vi "Open Drive Motors.vi"(5 "Open Butterfly Drive?":bool, 6 "Idle Mode":T1, 7 "Set Master/Follower?":bool, 9 "CAN IDs":u8[](array[numeric]), 11 "Full Acceleration Time":sgl) -> ()   [LabVIEW 2018]
uses:
  <vilib>/Rock Robotics/WPI/ThirdParty/REV Robotics/SPARK MAX/Typedef/Spark MAX Idle Mode.ctl
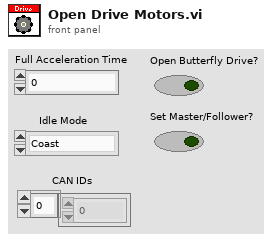
[diagram p1: front panel]
types:
  T1 = typedef "Spark MAX Idle Mode.ctl" = enum16{"Coast", "Brake"}
  T2 = typedef "WPI_MotorControlDeviceRef.ctl" = cluster{"DeviceStatus":errorcluster, "Type":T3, "PWM":cluster{"PWM Channel":T4, "DeadBand":T5}, "CAN":cluster{"Device Number":u8, "SetOutput VI Ref":variant, "GetOutput VI Ref":variant, "Enable VI Ref":variant, "Disable VI Ref":variant, "Data":variant}, "Invert":bool, "DIO PWM":cluster{"PWM \"Enable\" Channel":T4, "DIOChannel":T6, "PWM Rate":dbl}}
  T3 = typedef "WPI_MotorControlType.ctl" = enum16{"PWM", "CAN", "DIO PWM"}
  T4 = typedef "FPGA_DIOPWMChannel.ctl" = enum8{"PWM 0", "PWM 1", "PWM 2", "PWM 3", "PWM 4", "PWM 5", "PWM 6", "PWM 7", "PWM 8", "PWM 9", "PWM MXP 0", "PWM MXP 1", "PWM MXP 2", "PWM MXP 3", "PWM MXP 4", "PWM MXP 5", "PWM MXP 6", "PWM MXP 7", "PWM MXP 8", "PWM MXP 9", "Invalid"}
  T5 = typedef "WPI_PWMDeadband.ctl" = cluster{"Name":string, "maxPositivePwm":i32, "minPositivePwm":i32, "centerPwm":i32, "maxNegativePwm":i32, "minNegativePwm":i32, "angularRange":u16}
  T6 = typedef "FPGA_DIOChannel.ctl" = enum8{"DIO 0", "DIO 1", "DIO 2", "DIO 3", "DIO 4", "DIO 5", "DIO 6", "DIO 7", "DIO 8", "DIO 9", "DIO MXP 0", "DIO MXP 1", "DIO MXP 2", "DIO MXP 3", "DIO MXP 4", "DIO MXP 5", "DIO MXP 6", "DIO MXP 7", "DIO MXP 8", "DIO MXP 9", "DIO MXP 10", "DIO MXP 11", "DIO MXP 12", "DIO MXP 13", "DIO MXP 14", "DIO MXP 15", "SPI Port CS1", "SPI Port CS2", "SPI Port CS3", "SPI Port MISO", "SPI Port MOSI", "Invalid"}
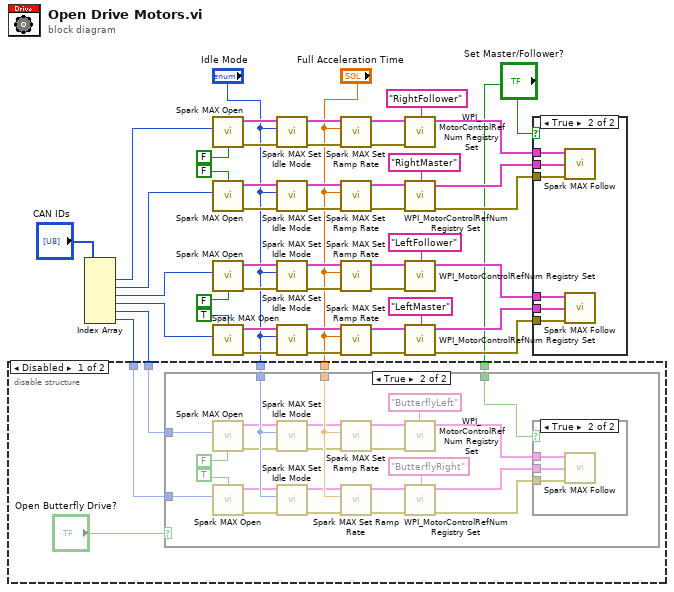
[diagram p0: block diagram]
diagram:
  n1 = Index Array(array="CAN IDs") -> (element #1=w10:u8, element #2=w9:u8, element #3=w8:u8, element #4=w7:u8, element #5=w6:u8, element #6=w5:u8)  [unwired: 6 in]
  n2 = disable-structure shown="Disabled" {
    disable-tunnel: w6 -> [w54 _]
    disable-tunnel: w5 -> [w53 _]
    disable-tunnel: "Full Acceleration Time" -> [w52 _]
    disable-tunnel: "Idle Mode" -> [w51 _]
    disable-tunnel: "Set Master/Follower?" -> [w49 _]
    frame Disabled {
      n3 = case shown="True" "Open Butterfly Drive?" {
        tunnel: w54 -> [_ w78]
        tunnel: w53 -> [_ w77]
        tunnel: w52 -> [_ w76]
        tunnel: w51 -> [_ w75]
        tunnel: w49 -> [_ w55]
        frame False {
        }
        frame True {
          n4 = call <vilib>:"Spark MAX Open.vi"("Invert"=FALSE, "Device Number"=w78) -> ("error out"=w59:errorcluster, "MotorControlDeviceRef"=w61:T2)  [unwired: 8 in]
          n5 = call <vilib>:"Spark MAX Open.vi"("Invert"=TRUE, "Device Number"=w77) -> ("error out"=w58:errorcluster, "MotorControlDeviceRef"=w60:T2)  [unwired: 8 in]
          n6 = call <vilib>:"Spark MAX Set Idle Mode.vi"("error in (no error)"=w59, "Idle Mode"=w75, "MotorControlDeviceRef in"=w61) -> ("error out"=w67:errorcluster, "MotorControlDeviceRef out"=w68:T2)  [unwired: 7 in]
          n7 = call <vilib>:"Spark MAX Set Idle Mode.vi"("error in (no error)"=w58, "Idle Mode"=w75, "MotorControlDeviceRef in"=w60) -> ("error out"=w65:errorcluster, "MotorControlDeviceRef out"=w69:T2)  [unwired: 7 in]
          n8 = call <vilib>:"Spark MAX Set Ramp Rate.vi"("error in (no error)"=w67, "Seconds from neutral to full (0)"=w76, "MotorControlDeviceRef in"=w68) -> ("error out"=w66:errorcluster, "MotorControlDeviceRef"=w70:T2)  [unwired: 7 in]
          n9 = call <vilib>:"Spark MAX Set Ramp Rate.vi"("error in (no error)"=w65, "Seconds from neutral to full (0)"=w76, "MotorControlDeviceRef in"=w69) -> ("error out"=w64:errorcluster, "MotorControlDeviceRef"=w71:T2)  [unwired: 7 in]
          n10 = call <vilib>:"WPI_MotorControlRefNum Registry Set.vi"("error in (no error)"=w66, "refnum name"="ButterflyLeft", "MotorControlDevRef"=w70) -> ("MotorControlDevRef"=w74:T2)  [unwired: 7 in, 1 out]
          n11 = call <vilib>:"WPI_MotorControlRefNum Registry Set.vi"("error in (no error)"=w64, "refnum name"="ButterflyRight", "MotorControlDevRef"=w71) -> ("error out"=w72:errorcluster, "MotorControlDevRef"=w73:T2)  [unwired: 7 in]
          n12 = case shown="True" w55 {
            tunnel: w74 -> [_ w81]
            tunnel: w73 -> [_ w80]
            tunnel: w72 -> [_ w79]
            frame False {
            }
            frame True {
              n13 = call <vilib>:"Spark MAX Follow.vi"("error in (no error)"=w79, "Master Controller"=w80, "MotorControlDeviceRef"=w81) -> ()  [unwired: 7 in, 2 out]
            }
          }
        }
      }
    }
    frame Enabled {
    }
  }
  n14 = call <vilib>:"Spark MAX Open.vi"("Invert"=FALSE, "Device Number"=w10) -> ("error out"=w35:errorcluster, "MotorControlDeviceRef"=w40:T2)  [unwired: 8 in]
  n15 = call <vilib>:"Spark MAX Open.vi"("Invert"=FALSE, "Device Number"=w9) -> ("error out"=w33:errorcluster, "MotorControlDeviceRef"=w39:T2)  [unwired: 8 in]
  n16 = call <vilib>:"Spark MAX Open.vi"("Invert"=FALSE, "Device Number"=w8) -> ("error out"=w31:errorcluster, "MotorControlDeviceRef"=w41:T2)  [unwired: 8 in]
  n17 = call <vilib>:"Spark MAX Open.vi"("Invert"=TRUE, "Device Number"=w7) -> ("error out"=w29:errorcluster, "MotorControlDeviceRef"=w42:T2)  [unwired: 8 in]
  n18 = call <vilib>:"Spark MAX Set Idle Mode.vi"("error in (no error)"=w35, "Idle Mode"="Idle Mode", "MotorControlDeviceRef in"=w40) -> ("error out"=w34:errorcluster, "MotorControlDeviceRef out"=w37:T2)  [unwired: 7 in]
  n19 = call <vilib>:"Spark MAX Set Idle Mode.vi"("error in (no error)"=w33, "Idle Mode"="Idle Mode", "MotorControlDeviceRef in"=w39) -> ("error out"=w32:errorcluster, "MotorControlDeviceRef out"=w38:T2)  [unwired: 7 in]
  n20 = call <vilib>:"Spark MAX Set Idle Mode.vi"("error in (no error)"=w31, "Idle Mode"="Idle Mode", "MotorControlDeviceRef in"=w41) -> ("error out"=w26:errorcluster, "MotorControlDeviceRef out"=w44:T2)  [unwired: 7 in]
  n21 = call <vilib>:"Spark MAX Set Idle Mode.vi"("error in (no error)"=w29, "Idle Mode"="Idle Mode", "MotorControlDeviceRef in"=w42) -> ("error out"=w28:errorcluster, "MotorControlDeviceRef out"=w43:T2)  [unwired: 7 in]
  n22 = call <vilib>:"Spark MAX Set Ramp Rate.vi"("error in (no error)"=w34, "Seconds from neutral to full (0)"="Full Acceleration Time", "MotorControlDeviceRef in"=w37) -> ("error out"=w24:errorcluster, "MotorControlDeviceRef"=w46:T2)  [unwired: 7 in]
  n23 = call <vilib>:"Spark MAX Set Ramp Rate.vi"("error in (no error)"=w32, "Seconds from neutral to full (0)"="Full Acceleration Time", "MotorControlDeviceRef in"=w38) -> ("error out"=w25:errorcluster, "MotorControlDeviceRef"=w45:T2)  [unwired: 7 in]
  n24 = call <vilib>:"Spark MAX Set Ramp Rate.vi"("error in (no error)"=w26, "Seconds from neutral to full (0)"="Full Acceleration Time", "MotorControlDeviceRef in"=w44) -> ("error out"=w30:errorcluster, "MotorControlDeviceRef"=w47:T2)  [unwired: 7 in]
  n25 = call <vilib>:"Spark MAX Set Ramp Rate.vi"("error in (no error)"=w28, "Seconds from neutral to full (0)"="Full Acceleration Time", "MotorControlDeviceRef in"=w43) -> ("error out"=w27:errorcluster, "MotorControlDeviceRef"=w48:T2)  [unwired: 7 in]
  n26 = call <vilib>:"WPI_MotorControlRefNum Registry Set.vi"("error in (no error)"=w24, "refnum name"="RightFollower" ("string"), "MotorControlDevRef"=w46) -> ("MotorControlDevRef"=w18:T2)  [unwired: 7 in, 1 out]
  n27 = call <vilib>:"WPI_MotorControlRefNum Registry Set.vi"("error in (no error)"=w25, "refnum name"="RightMaster", "MotorControlDevRef"=w45) -> ("error out"=w2:errorcluster, "MotorControlDevRef"=w17:T2)  [unwired: 7 in]
  n28 = call <vilib>:"WPI_MotorControlRefNum Registry Set.vi"("error in (no error)"=w30, "refnum name"="LeftFollower", "MotorControlDevRef"=w47) -> ("MotorControlDevRef"=w14:T2)  [unwired: 7 in, 1 out]
  n29 = call <vilib>:"WPI_MotorControlRefNum Registry Set.vi"("error in (no error)"=w27, "refnum name"="LeftMaster", "MotorControlDevRef"=w48) -> ("error out"=w20:errorcluster, "MotorControlDevRef"=w16:T2)  [unwired: 7 in]
  n30 = case shown="True" "Set Master/Follower?" {
    tunnel: w20 -> [_ w87]
    tunnel: w18 -> [_ w86]
    tunnel: w17 -> [_ w85]
    tunnel: w16 -> [_ w84]
    tunnel: w14 -> [_ w83]
    tunnel: w2 -> [_ w82]
    frame False {
    }
    frame True {
      n31 = call <vilib>:"Spark MAX Follow.vi"("error in (no error)"=w82, "Master Controller"=w85, "MotorControlDeviceRef"=w86) -> ()  [unwired: 7 in, 2 out]
      n32 = call <vilib>:"Spark MAX Follow.vi"("error in (no error)"=w87, "Master Controller"=w84, "MotorControlDeviceRef"=w83) -> ()  [unwired: 7 in, 2 out]
    }
  }
